vi "改动项处理模块.vi"(6 "执行模式":enum16{"连接模式", "离线模式"}(ring), 7 "改动项 i":T2, 9 "串口配置":T1, 10 "探头属性 i":T7, 11 "TCP ID i":refnum<k5>) -> (0 "error out":errorcluster, 2 "探头属性 o":T7, 3 "TCP ID o":refnum<k5>, 5 "改动项复位 o":T2)   [LabVIEW 2017]
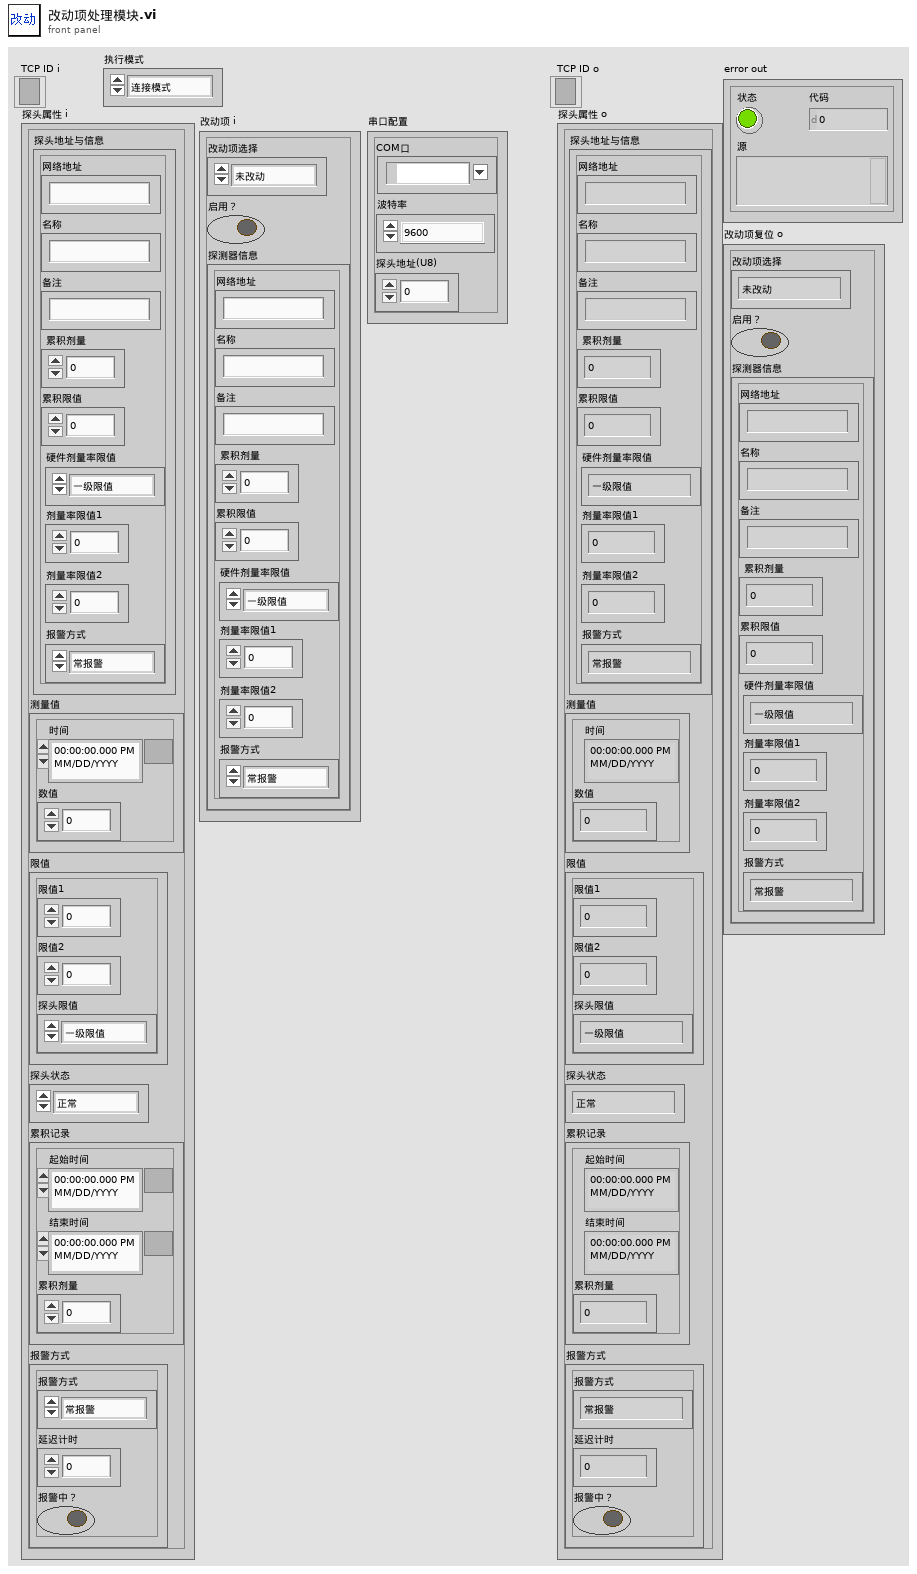
[diagram p1: front panel]
types:
  T1 = typedef "串口配置.ctl" = cluster{"COM口":refnum<visa-resource-name>, "波特率":enum16{"9600", "19200"}, "探头地址(U8)":u8}
  T2 = typedef "改动项.ctl" = cluster{"改动项选择":T3, "启用？":bool, "探测器信息":T4}
  T3 = typedef "改动项选择.ctl" = enum16{"未改动", "改动-启用状态", "改动-探头信息", "改动-报警限值", "动作-手动静音", "动作-重启累积时段", "动作-累积删除", "动作-重连"}
  T4 = typedef "探测器信息.ctl" = cluster{"网络地址":string, "名称":string, "备注":string, "累积剂量":dbl, "累积限值":dbl, "硬件剂量率限值":T5, "剂量率限值1":dbl, "剂量率限值2":dbl, "报警方式":T6}
  T5 = typedef "探头剂量率限值选择.ctl" = enum16{"一级限值", "二级限值"}
  T6 = typedef "报警方式选择.ctl" = enum16{"常报警", "自动静音", "手动静音"}
  T7 = typedef "探头属性.ctl" = cluster{"探头地址与信息":T4, "测量值":T8, "限值":T9, "探头状态":T10, "累积记录":T11, "报警方式":T12}
  T8 = typedef "测量值.ctl" = cluster{"时间":timestamp, "数值":dbl}
  T9 = typedef "剂量率限值.ctl" = cluster{"限值1":dbl, "限值2":dbl, "探头限值":T5}
  T10 = typedef "探头状态.ctl" = enum16{"正常", "离线", "禁用", "一级报警", "二级报警", "累积报警"}
  T11 = typedef "单条累积记录.ctl" = cluster{"起始时间":timestamp, "结束时间":timestamp, "累积剂量":dbl}
  T12 = typedef "报警方式.ctl" = cluster{"报警方式":T6, "延迟计时":u16, "报警中？":bool}
  T13 = typedef "串口模块输入.ctl" = cluster{"串口动作类型":T14, "串口配置":T1, "数据输入":variant}
  T14 = typedef "串口动作类型.ctl" = enum16{"读测量值", "设置报警值", "设置地址", "设置系数", "广播修改波特率", "关闭串口"}
  T15 = typedef "DB动作与数据.ctl" = cluster{"动作类型":T16, "输入数据":variant}
  T16 = typedef "DB动作类型.ctl" = enum16{"DB-文件初始化+连接", "DB-断开连接", "DB-结构初始化", "DB-加载设备", "DB-检查连接状态", "设备-登记新设备+数据表", "设备-删除设备", "设备-修改网址", "设备-修改名称+转移数据", "设备-修改备注", "设备-修改限值", "设备-累积校准", "设备-重排", "数据-获取全部", "数据-删除数据", "数据-写改累积记录+改累积剂量", "读变量-全部设备"}
  T17 = typedef "设备改名卡.ctl" = cluster{"原名":string, "新名":string}
  T18 = typedef "修改网址.ctl" = cluster{"探头属性":T4, "新网址":string}
  T19 = typedef "删除记录输入.ctl" = cluster{"名称":string, "多条记录(空则全删)":T11[]}
  T20 = cluster{"网络地址":bool, "名称":bool, "备注":bool, "累积剂量":bool, "累积限值":bool, "硬件剂量率限值":bool, "剂量率限值1":bool, "剂量率限值2":bool, "报警方式":bool}
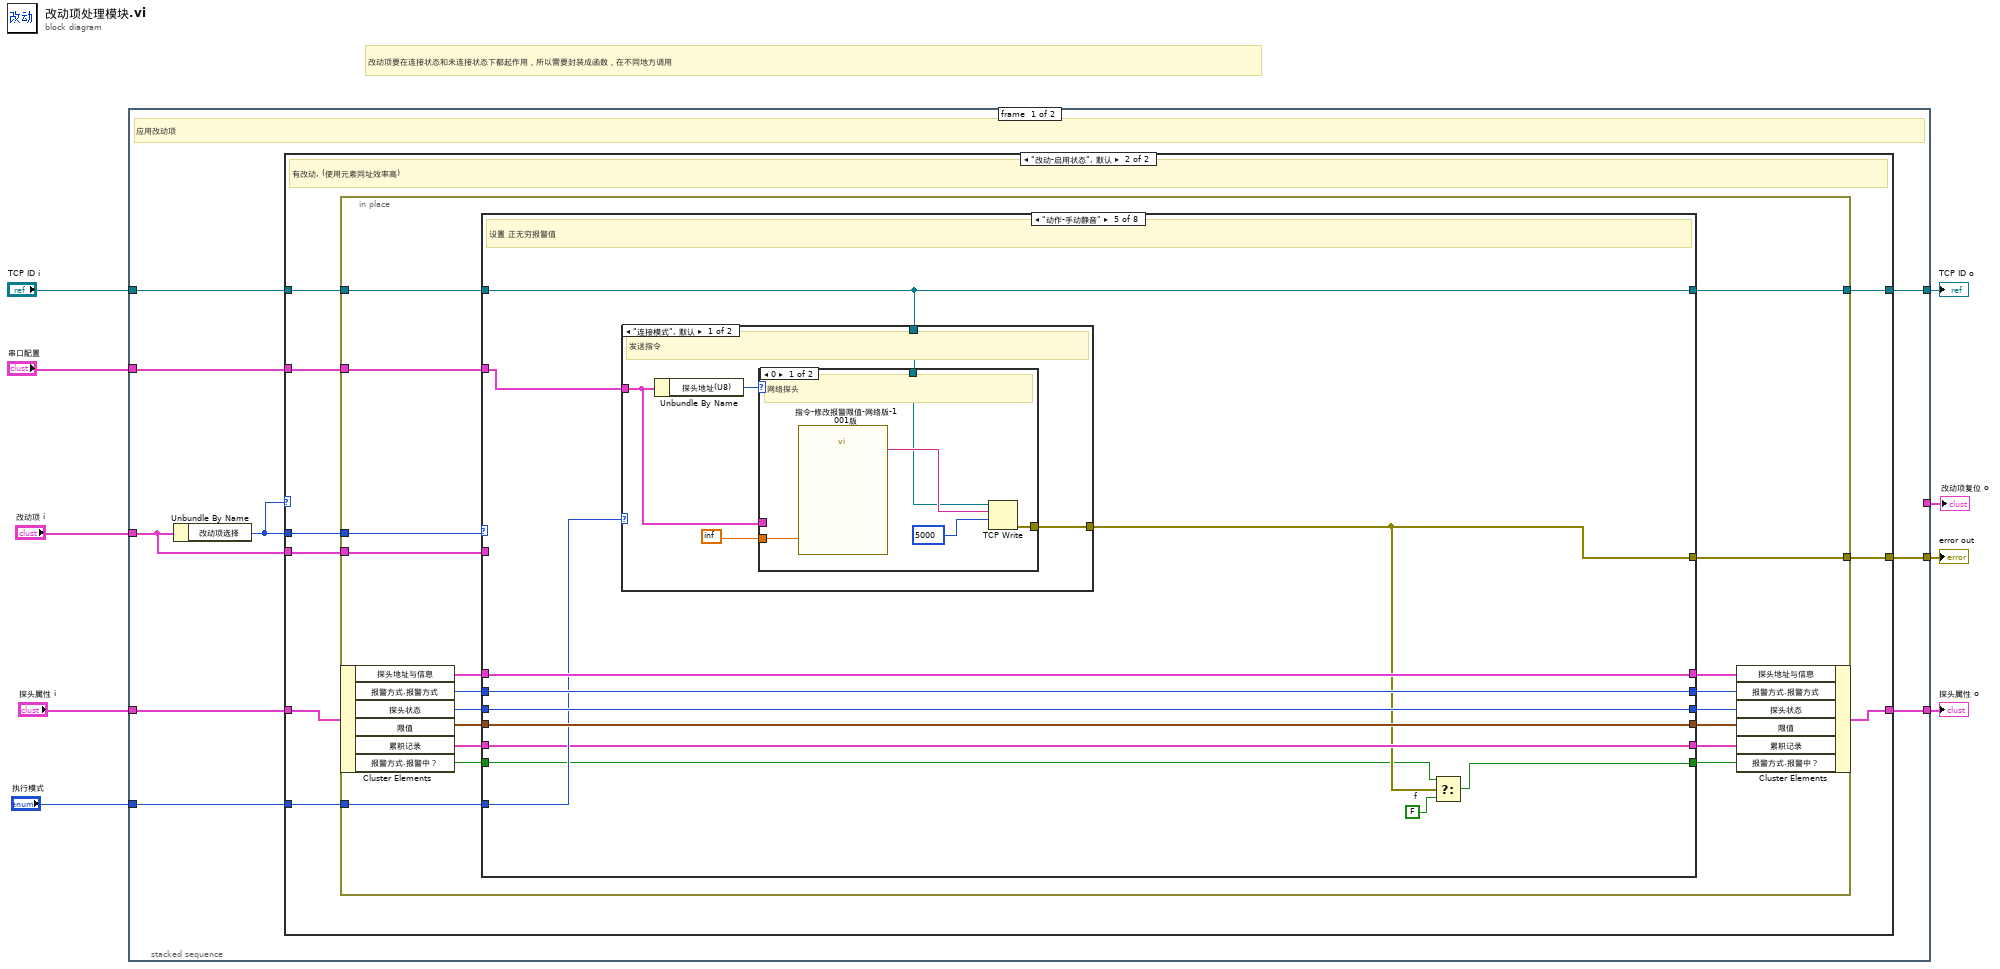
[diagram p0: block diagram]
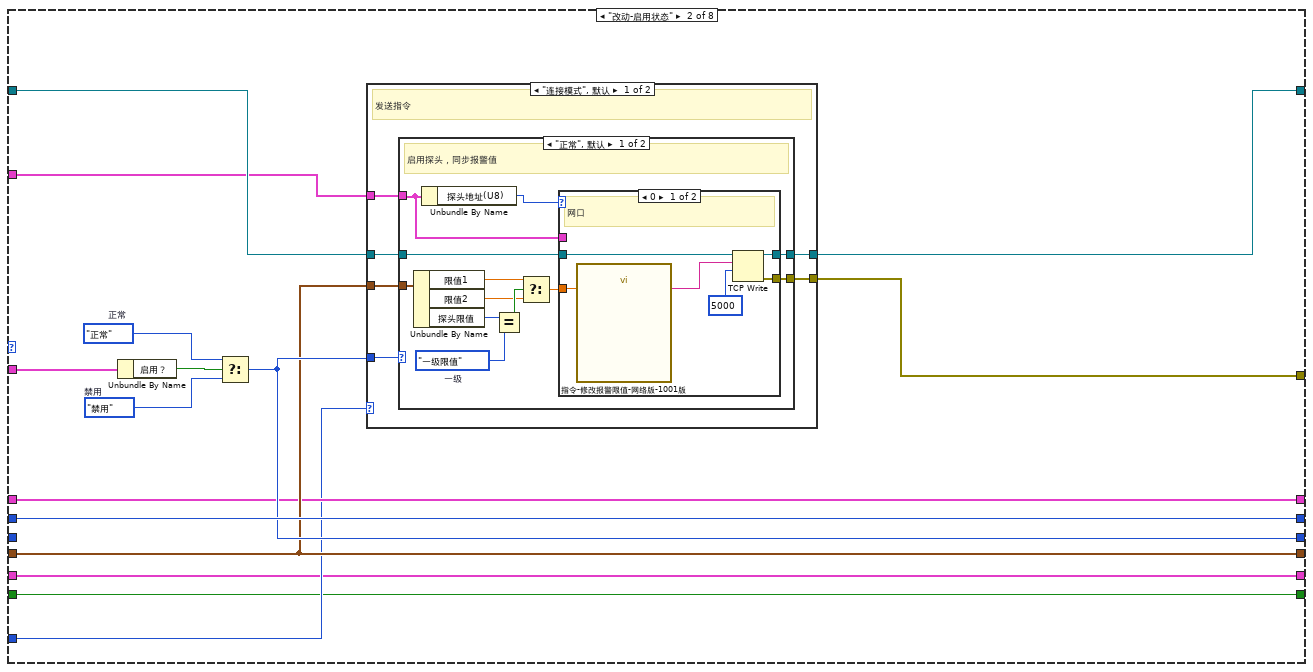
[diagram p4: hidden frame]
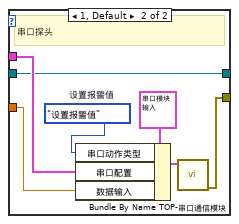
[diagram p5: hidden frame]
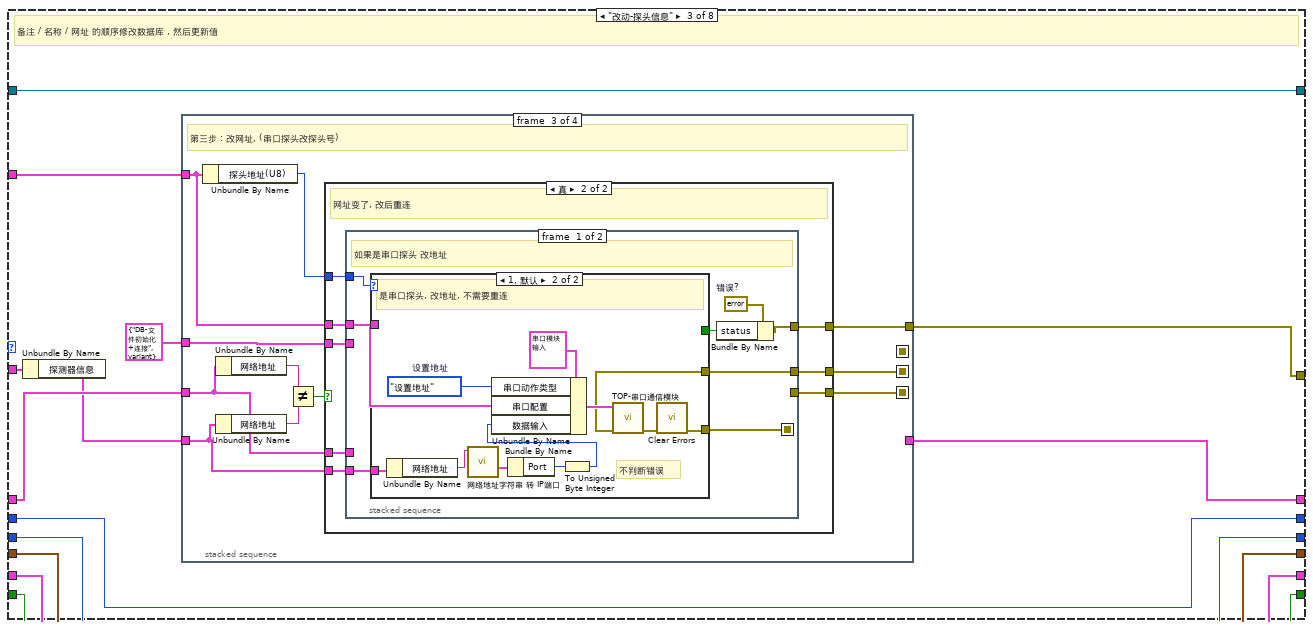
[diagram p8: hidden frame]
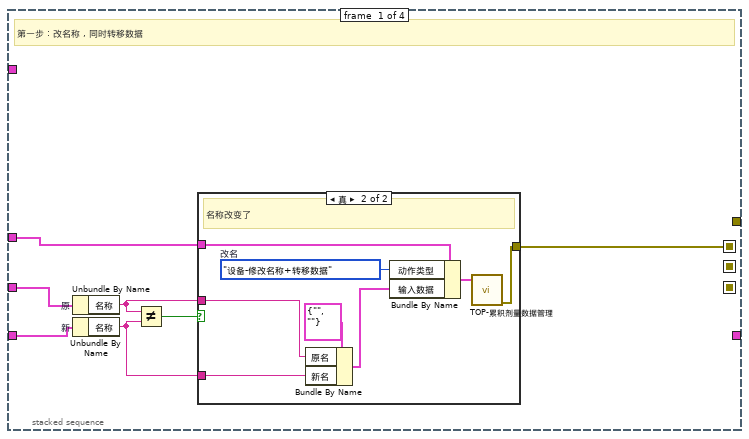
[diagram p9: hidden frame]
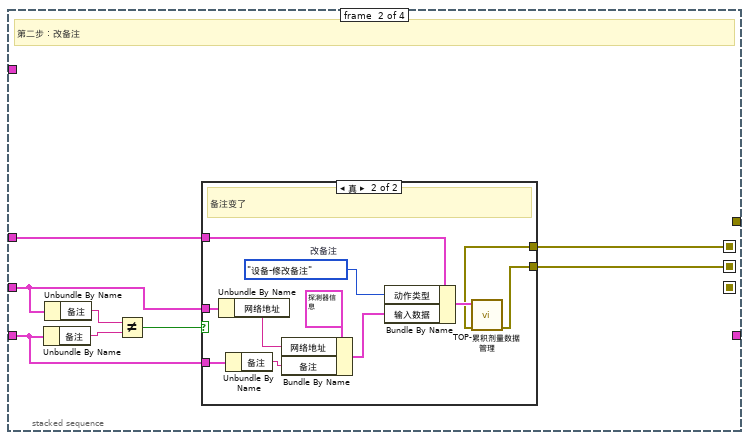
[diagram p11: hidden frame]
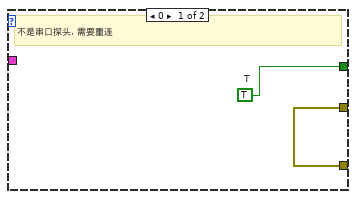
[diagram p14: hidden frame]
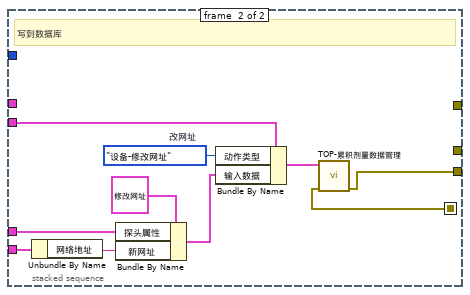
[diagram p15: hidden frame]
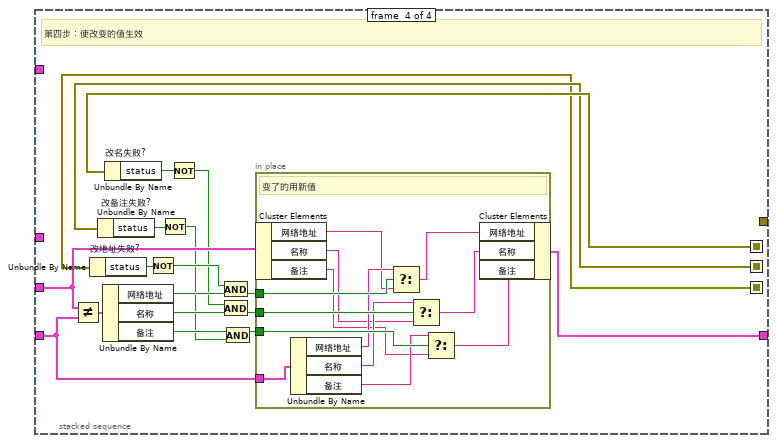
[diagram p16: hidden frame]
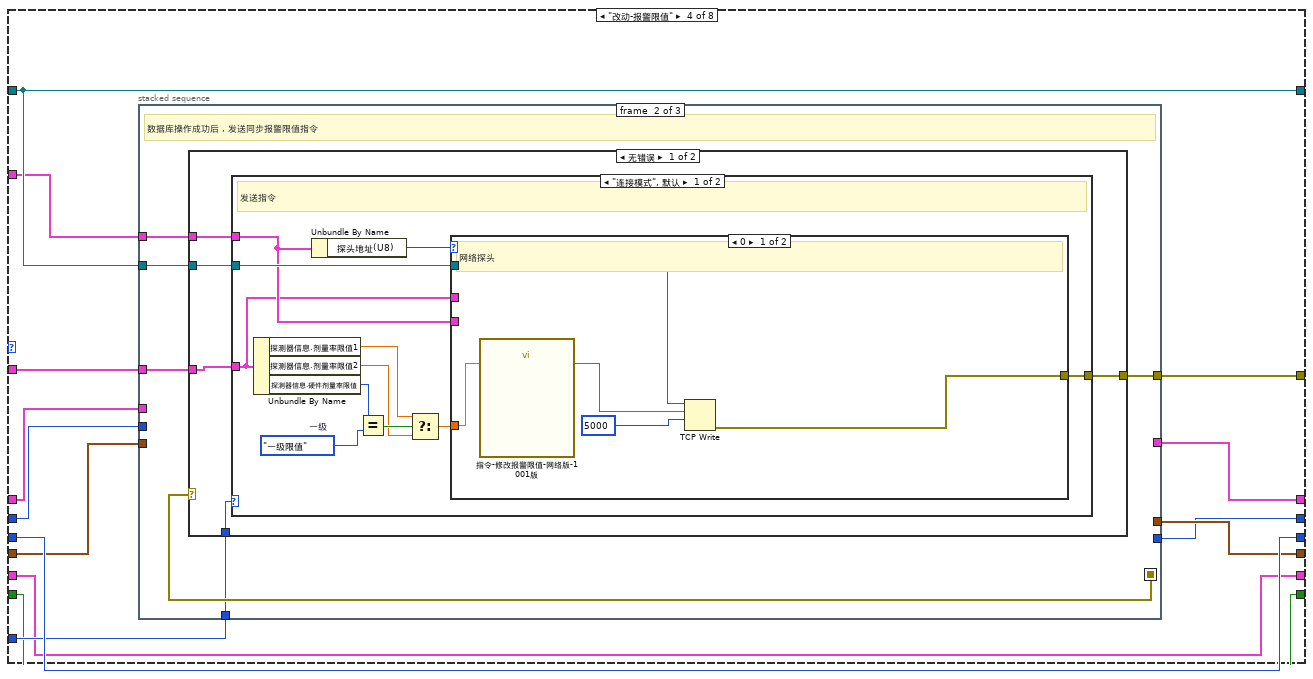
[diagram p17: hidden frame]
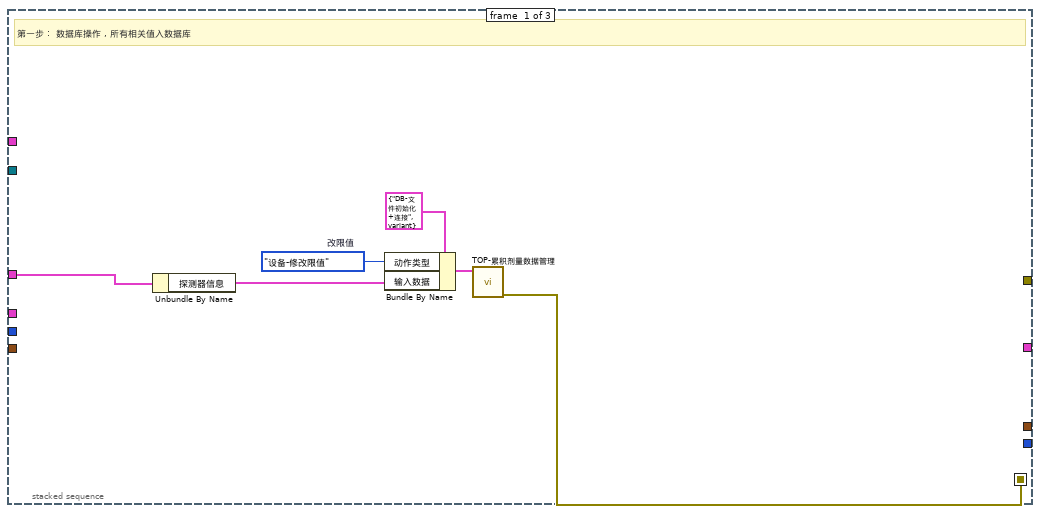
[diagram p18: hidden frame]
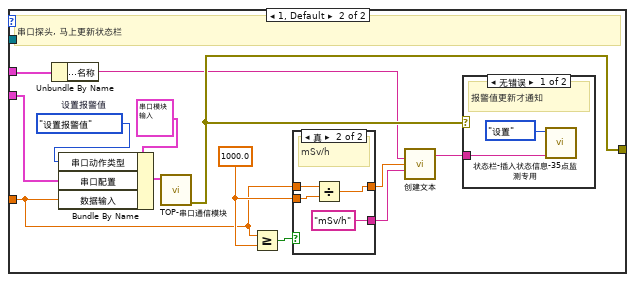
[diagram p19: hidden frame]
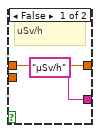
[diagram p20: hidden frame]
diagram:
  # "改动项要在连接状态和未连接状态下都起作用，所以需要封装成函数，在不同地方调用"
  n1 = stacked-sequence {
    tunnel: "改动项 i" -> [w12 _]
    tunnel: [w18 _] -> w5
    tunnel: "探头属性 i" -> [w17 _]
    tunnel: "TCP ID i" -> [w16 _]
    tunnel: [w15 _] -> w4
    tunnel: [w14 _] -> w7
    tunnel: [_ T2 {"改动项选择"=enum."未改动", "启用？"=FALSE, "探测器信息"={"网络地址"="", "名称"="", "备注"="", "累积剂量"=0.0, "累积限值"=0.0, "硬件剂量率限值"=enum."一级限值", "剂量率限值1"=0.0, "剂量率限值2"=0.0, "报警方式"=enum."常报警"}} ("改动项")] -> w3
    tunnel: "执行模式" -> [w13 _]
    tunnel: "串口配置" -> [w10 _]
    frame #0 {
      # "应用改动项"
      n2 = Unbundle By Name(w12) -> ("改动项选择"=w11:T3)
      n3 = case shown="\"改动-启用状态\", 默认" w11 {
        tunnel: w11 -> [_ w29]
        tunnel: [w19 w28] -> w18
        tunnel: w17 -> [w19 w27]
        tunnel: w16 -> [w20 w26]
        tunnel: [_ w25] -> w15
        tunnel: [w20 w24] -> w14
        tunnel: w13 -> [_ w23]
        tunnel: w12 -> [_ w22]
        tunnel: w10 -> [_ w21]
        frame "未改动" {
          # "未改动就不操作"
        }
        frame "改动-启用状态", Default {
          # "有改动, (使用元素同址效率高)"
          n4 = in-place {
            in-place-border: w29 -> [w48]
            in-place-border: w26 -> [w41]
            in-place-border: [w40] -> w24
            in-place-border: [w39] -> w25
            in-place-border: w23 -> [w36]
            in-place-border: w22 -> [w32]
            in-place-border: w21 -> [w33]
            n5 = in-place-cluster #1(w27) -> ("探头地址与信息"=w37:T4, "报警方式.报警方式"=w46:T6, "探头状态"=w45:T10, "限值"=w43:T9, "累积记录"=w35:T11, "报警方式.报警中？"=w31:bool)
            n6 = case shown="\"动作-手动静音\"" w48 {
              tunnel: w32 -> [_ w70 w116 w248 _ _ w382 _]
              tunnel: [w55 w66 w108 w242 w342 w369 w378 w404] -> w47
              tunnel: w46 -> [w55 w66 w108 w240 w342 w369 w378 w404]
              tunnel: [w54 w65 w113 w249 w343 w368 w379 w403] -> w44
              tunnel: w45 -> [w54 _ w113 w249 w343 w368 w379 w403]
              tunnel: w43 -> [w53 w62 w114 w245 w344 w367 w380 w402]
              tunnel: [w53 w62 w114 w243 w344 w367 w380 w402] -> w42
              tunnel: w41 -> [w52 w64 w112 w247 w340 w366 w386 w400]
              tunnel: [w52 w63 w112 w247 w340 w366 w386 w400] -> w40
              tunnel: [_ w57 w107 w246 w335 _ _ w407] -> w39
              tunnel: [w51 w61 w109 w241 w341 w370 w385 w405] -> w38
              tunnel: w37 -> [w51 w61 w115 w244 w341 w370 w372 w405]
              tunnel: w36 -> [_ w60 _ w239 w339 _ _ _]
              tunnel: w35 -> [w50 w59 w106 w238 w338 w365 w375 w401]
              tunnel: [w50 w59 w106 w238 w338 w362 w374 w401] -> w34
              tunnel: w33 -> [_ w58 w105 w237 w337 _ _ _]
              tunnel: w31 -> [w49 w56 w104 w236 w334 w361 w371 w399]
              tunnel: [w49 w56 w104 w236 w333 w361 w371 w399] -> w30
              frame "未改动", Default {
                # "未改动"
              }
              frame "改动-启用状态" {
                w68 = 探头状态."禁用"  # 禁用
                w67 = 探头状态."正常"  # 正常
                n7 = Unbundle By Name(w70) -> ("启用？"=w69:bool)
                n8 = Select(t=w67, s=w69, f=w68) -> (s? t:f=w65:T10)
                n9 = case shown="\"连接模式\", 默认" w60 {
                  tunnel: w65 -> [w76 _]
                  tunnel: w64 -> [w75 w103]
                  tunnel: [w74 w103] -> w63
                  tunnel: w62 -> [w73 _]
                  tunnel: [w72 _] -> w57
                  tunnel: w58 -> [w71 _]
                  frame "连接模式", Default {
                    # "发送指令"
                    n10 = case shown="\"正常\", 默认" w76 {
                      tunnel: w73 -> [w88 _]
                      tunnel: w75 -> [w87 w102]
                      tunnel: [w86 w102] -> w74
                      tunnel: [w85 _] -> w72
                      tunnel: w71 -> [w77 _]
                      frame "正常", Default {
                        w83 = 探头剂量率限值选择."一级限值"  # 一级
                        # "启用探头，同步报警值"
                        n11 = Unbundle By Name(w88) -> ("限值1"=w80:dbl, "限值2"=w81:dbl, "探头限值"=w84:T5)
                        n12 = Unbundle By Name(w77) -> ("探头地址(U8)"=w78:u8)
                        n13 = Equal?(x=w84, y=w83) -> (x = y?=w82:bool)
                        n14 = Select(t=w80, s=w82, f=w81) -> (s? t:f=w79:dbl)
                        n15 = case shown="0" w78 {
                          tunnel: w87 -> [w92 w95]
                          tunnel: [w91 w95] -> w86
                          tunnel: [w90 w96] -> w85
                          tunnel: w79 -> [w89 w97]
                          tunnel: w77 -> [_ w98]
                          frame 0 {
                            # "网口"
                            n16 = call "指令-修改报警限值-网络版-1001版.vi"("限值"=w89) -> ("指令输出"=w93:string)  [unwired: 10 in]
                            n17 = TCP Write(connection ID=w92, data in=w93, 9:5000 ("超时毫秒(25000)")) -> (connection ID out=w91:refnum<k5>, error out=w90:errorcluster)  [unwired: 1 in, 1 out]
                          }
                          frame 1, Default {
                            w101 = 串口动作类型."设置报警值"  # 设置报警值
                            # "串口探头"
                            n18 = Bundle By Name(cluster=T13 {"串口动作类型"=enum."读测量值", "串口配置"={"COM口"="", "波特率"=enum."9600", "探头地址(U8)"=0}, "数据输入"=variant} ("串口模块输入"), "串口动作类型"=w101, "串口配置"=w98, "数据输入"=w97) -> (w100:T13)
                            n19 = call "TOP-串口通信模块.vi"("串口模块输入"=w100) -> ("error out"=w96:errorcluster)  [unwired: 9 in, 1 out]
                          }
                        }
                      }
                      frame "禁用" {
                      }
                    }
                  }
                  frame "离线模式" {
                    # "不发送指令"
                  }
                }
              }
              frame "改动-探头信息" {
                # "备注 / 名称 / 网址 的顺序修改数据库 , 然后更新值"
                n20 = Unbundle By Name(w116) -> ("探测器信息"=w110:T4)
                n21 = stacked-sequence {
                  seq-local: [w122 _ _ _] -> [_ w137 _ w212]
                  seq-local: [_ w138 _ _] -> [_ _ w161 w211]
                  seq-local: [_ _ w155 _] -> [_ _ _ w210]
                  tunnel: w115 -> [w121 w136 w160 w221]
                  tunnel: T15 {"动作类型"=enum."DB-文件初始化+连接", "输入数据"=variant} ("DB动作集") -> [w123 w139 w162 _]
                  tunnel: w110 -> [w120 w135 w159 w217]
                  tunnel: [_ _ _ w216] -> w109
                  tunnel: [_ _ w154 _] -> w107
                  tunnel: w105 -> [_ _ w152 _]
                  frame #0 {
                    # "第一步 : 改名称 , 同时转移数据"
                    n22 = Unbundle By Name "原"(w121) -> ("名称"=w118:string)
                    n23 = Unbundle By Name "新"(w120) -> ("名称"=w117:string)
                    n24 = Not Equal?(x=w118, y=w117) -> (x != y?=w119:bool)
                    n25 = case shown="真" w119 {
                      tunnel: w123 -> [_ w131]
                      tunnel: [_ w126] -> w122
                      tunnel: w118 -> [_ w125]
                      tunnel: w117 -> [_ w124]
                      frame False {
                        # "名称没变"
                      }
                      frame True {
                        w130 = DB动作类型."设备-修改名称+转移数据"  # 改名
                        # "名称改变了"
                        n26 = Bundle By Name(cluster=T17 {"原名"="", "新名"=""} ("改名"), "原名"=w125, "新名"=w124) -> (w128:T17)
                        n27 = Bundle By Name(cluster=w131, "动作类型"=w130, "输入数据"=w128) -> (w127:T15)
                        n28 = call "TOP-累积剂量数据管理.vi"("DB动作集"=w127) -> ("error out"=w126:errorcluster)  [unwired: 9 in, 1 out]
                      }
                    }
                  }
                  frame #1 {
                    # "第二步 : 改备注"
                    n29 = Unbundle By Name(w135) -> ("备注"=w133:string)
                    n30 = Unbundle By Name(w136) -> ("备注"=w134:string)
                    n31 = Not Equal?(x=w134, y=w133) -> (x != y?=w132:bool)
                    n32 = case shown="真" w132 {
                      tunnel: w139 -> [_ w150]
                      tunnel: [w140 w144] -> w138
                      tunnel: w137 -> [w140 w143]
                      tunnel: w136 -> [_ w142]
                      tunnel: w135 -> [_ w141]
                      frame False {
                        # "备注没变"
                      }
                      frame True {
                        w151 = DB动作类型."设备-修改备注"  # 改备注
                        # "备注变了"
                        n33 = Unbundle By Name(w142) -> ("网络地址"=w147:string)
                        n34 = Unbundle By Name(w141) -> ("备注"=w148:string)
                        n35 = Bundle By Name(cluster=T4 {"网络地址"="", "名称"="", "备注"="", "累积剂量"=0.0, "累积限值"=0.0, "硬件剂量率限值"=enum."一级限值", "剂量率限值1"=0.0, "剂量率限值2"=0.0, "报警方式"=enum."常报警"} ("探测器信息-改备注"), "网络地址"=w147, "备注"=w148) -> (w146:T4)
                        n36 = Bundle By Name(cluster=w150, "动作类型"=w151, "输入数据"=w146) -> (w145:T15)
                        n37 = call "TOP-累积剂量数据管理.vi"("错误输出"=w143, "DB动作集"=w145) -> ("error out"=w144:errorcluster)  [unwired: 8 in, 1 out]
                      }
                    }
                  }
                  frame #2 {
                    # "第三步 : 改网址, (串口探头改探头号)"
                    n38 = Unbundle By Name(w152) -> ("探头地址(U8)"=w153:u8)
                    n39 = Unbundle By Name(w160) -> ("网络地址"=w158:string)
                    n40 = Unbundle By Name(w159) -> ("网络地址"=w157:string)
                    n41 = Not Equal?(x=w158, y=w157) -> (x != y?=w156:bool)
                    n42 = case shown="真" w156 {
                      tunnel: w162 -> [_ w167]
                      tunnel: w161 -> [w163 w171]
                      tunnel: w160 -> [_ w170]
                      tunnel: w159 -> [_ w169]
                      tunnel: [w163 w168] -> w155
                      tunnel: [_ w166] -> w154
                      tunnel: w153 -> [_ w165]
                      tunnel: w152 -> [_ w164]
                      frame False {
                        # "网址没变"
                      }
                      frame True {
                        # "网址变了, 改后重连"
                        n43 = stacked-sequence {
                          seq-local: [w172 _] -> [_ w194]
                          tunnel: w171 -> [w173 _]
                          tunnel: w170 -> [_ w198]
                          tunnel: w169 -> [w177 w197]
                          tunnel: [_ w196] -> w168
                          tunnel: w167 -> [_ w195]
                          tunnel: [w175 _] -> w166
                          tunnel: w165 -> [w179 _]
                          tunnel: w164 -> [w178 _]
                          frame #0 {
                            w176 = errorcluster {"status"=TRUE, "code"=0, "source"=""}  # 错误?
                            # "如果是串口探头 改地址"
                            n44 = case shown="1, 默认" w179 {
                              tunnel: w178 -> [_ w186]
                              tunnel: w177 -> [_ w191]
                              tunnel: [w181 _] -> w174
                              tunnel: w173 -> [w180 w184]
                              tunnel: [w180 w182] -> w172
                              frame 0 {
                                w181 = TRUE  # T
                                # "不是串口探头, 需要重连"
                              }
                              frame 1, Default {
                                w192 = 串口动作类型."设置地址"  # 设置地址
                                # "不判断错误"
                                # "是串口探头, 改地址, 不需要重连"
                                n45 = Unbundle By Name(w191) -> ("网络地址"=w189:string)
                                n46 = call "网络地址字符串 转 IP端口.vi"("IP端口字符串"=w189) -> ("IP端口"=w190:cluster{"IP":string, "Port":u16})  [unwired: 10 in]
                                n47 = Unbundle By Name(w190) -> ("Port"=w188:u16)
                                n48 = To Unsigned Byte Integer(number=w188) -> (unsigned 8bit integer=w187:u8)
                                n49 = Bundle By Name(cluster=T13 {"串口动作类型"=enum."读测量值", "串口配置"={"COM口"="", "波特率"=enum."9600", "探头地址(U8)"=0}, "数据输入"=variant} ("串口模块输入"), "串口动作类型"=w192, "串口配置"=w186, "数据输入"=w187) -> (w185:T13)
                                n50 = call "TOP-串口通信模块.vi"("错误输入（无错误）"=w184, "串口模块输入"=w185) -> ("error out"=w183:errorcluster)  [unwired: 8 in, 1 out]
                                n51 = call <vilib>:"Clear Errors.vi"("error in (no error)"=w183) -> ("error out"=w182:errorcluster)  [unwired: 5 in, 1 out]
                              }
                            }
                            n52 = Bundle By Name(cluster=w176, "status"=w174) -> (w175:errorcluster)
                          }
                          frame #1 {
                            w203 = DB动作类型."设备-修改网址"  # 改网址
                            # "写到数据库"
                            n53 = Unbundle By Name(w197) -> ("网络地址"=w201:string)
                            n54 = Bundle By Name(cluster=T18 {"探头属性"={"网络地址"="", "名称"="", "备注"="", "累积剂量"=0.0, "累积限值"=0.0, "硬件剂量率限值"=enum."一级限值", "剂量率限值1"=0.0, "剂量率限值2"=0.0, "报警方式"=enum."常报警"}, "新网址"=""} ("类型"), "探头属性"=w198, "新网址"=w201) -> (w200:T18)
                            n55 = Bundle By Name(cluster=w195, "动作类型"=w203, "输入数据"=w200) -> (w199:T15)
                            n56 = call "TOP-累积剂量数据管理.vi"("错误输出"=w194, "DB动作集"=w199) -> ("error out"=w196:errorcluster)  [unwired: 8 in, 1 out]
                          }
                        }
                      }
                    }
                  }
                  frame #3 {
                    # "第四步 : 使改变的值生效"
                    n57 = Not Equal?(x=w221, y=w217) -> (x != y?=w222:T20)
                    n58 = Unbundle By Name "改地址失败?"(w210) -> ("status"=w207:bool)
                    n59 = Unbundle By Name "改备注失败?"(w211) -> ("status"=w208:bool)
                    n60 = Unbundle By Name(w222) -> ("网络地址"=w220:bool, "名称"=w219:bool, "备注"=w218:bool)
                    n61 = Unbundle By Name "改名失败?"(w212) -> ("status"=w209:bool)
                    n62 = Not(x=w207) -> (.not. x?=w206:bool)
                    n63 = Not(x=w208) -> (.not. x?=w204:bool)
                    n64 = Not(x=w209) -> (.not. x?=w205:bool)
                    n65 = And(x=w206, y=w220) -> (x .and. y?=w215:bool)
                    n66 = And(x=w205, y=w219) -> (x .and. y?=w214:bool)
                    n67 = And(x=w218, y=w204) -> (x .and. y?=w213:bool)
                    n68 = in-place {
                      in-place-border: w215 -> [w235]
                      in-place-border: w214 -> [w234]
                      in-place-border: w213 -> [w233]
                      in-place-border: w217 -> [w232]
                      # "变了的用新值"
                      n69 = in-place-cluster #2(w221) -> ("网络地址"=w228:string, "名称"=w227:string, "备注"=w226:string)
                      n70 = Unbundle By Name(w232) -> ("网络地址"=w231:string, "名称"=w230:string, "备注"=w229:string)
                      n71 = Select(t=w231, s=w235, f=w228) -> (s? t:f=w225:string)
                      n72 = Select(t=w230, s=w234, f=w227) -> (s? t:f=w224:string)
                      n73 = Select(t=w229, s=w233, f=w226) -> (s? t:f=w223:string)
                      n74 = in-place-cluster #2("网络地址"=w225, "名称"=w224, "备注"=w223) -> (w216:T4)
                    }
                  }
                }
              }
              frame "改动-报警限值" {
                n75 = stacked-sequence {
                  seq-local: [w250 _ _] -> [_ w261 w311]
                  tunnel: w248 -> [w252 w260 w310]
                  tunnel: w247 -> [_ w259 _]
                  tunnel: [_ w258 _] -> w246
                  tunnel: w245 -> [_ _ w309]
                  tunnel: w244 -> [_ _ w308]
                  tunnel: [_ _ w307] -> w243
                  tunnel: [_ _ w306] -> w242
                  tunnel: [_ _ w305] -> w241
                  tunnel: w240 -> [_ _ w304]
                  tunnel: w239 -> [_ w257 _]
                  tunnel: w237 -> [_ w256 _]
                  frame #0 {
                    w255 = DB动作类型."设备-修改限值"  # 改限值
                    # "第一步 :  数据库操作 , 所有相关值入数据库"
                    n76 = Unbundle By Name(w252) -> ("探测器信息"=w251:T4)
                    n77 = Bundle By Name(cluster=T15 {"动作类型"=enum."DB-文件初始化+连接", "输入数据"=variant} ("DB动作集"), "动作类型"=w255, "输入数据"=w251) -> (w254:T15)
                    n78 = call "TOP-累积剂量数据管理.vi"("DB动作集"=w254) -> ("error out"=w250:errorcluster)  [unwired: 9 in, 1 out]
                  }
                  frame #1 {
                    # "数据库操作成功后 , 发送同步报警限值指令"
                    n79 = case shown="无错误" w261 {
                      tunnel: w260 -> [w266 _]
                      tunnel: w259 -> [w265 _]
                      tunnel: [w264 _] -> w258
                      tunnel: w257 -> [w263 _]
                      tunnel: w256 -> [w262 _]
                      frame No Error {
                        n80 = case shown="\"连接模式\", 默认" w263 {
                          tunnel: w266 -> [w267 _]
                          tunnel: w265 -> [w271 _]
                          tunnel: [w270 _] -> w264
                          tunnel: w262 -> [w268 _]
                          frame "连接模式", Default {
                            w276 = 探头剂量率限值选择."一级限值"  # 一级
                            # "发送指令"
                            n81 = Unbundle By Name(w267) -> ("探测器信息.剂量率限值1"=w274:dbl, "探测器信息.剂量率限值2"=w273:dbl, "探测器信息.硬件剂量率限值"=w277:T5)
                            n82 = Unbundle By Name(w268) -> ("探头地址(U8)"=w269:u8)
                            n83 = Equal?(x=w277, y=w276) -> (x = y?=w275:bool)
                            n84 = Select(t=w274, s=w275, f=w273) -> (s? t:f=w272:dbl)
                            n85 = case shown="0" w269 {
                              tunnel: w272 -> [w280 w285]
                              tunnel: w271 -> [w279 _]
                              tunnel: [w278 w290] -> w270
                              tunnel: w268 -> [_ w292]
                              tunnel: w267 -> [_ w289]
                              frame 0 {
                                # "网络探头"
                                n86 = call "指令-修改报警限值-网络版-1001版.vi"("限值"=w280) -> ("指令输出"=w282:string)  [unwired: 10 in]
                                n87 = TCP Write(connection ID=w279, data in=w282, 9:5000 ("超时毫秒(25000)")) -> (error out=w278:errorcluster)  [unwired: 1 in, 2 out]
                              }
                              frame 1, Default {
                                w286 = 1000.0 ("y")
                                w293 = 串口动作类型."设置报警值"  # 设置报警值
                                # "串口探头, 马上更新状态栏"
                                n88 = Unbundle By Name(w289) -> ("探测器信息.名称"=w288:string)
                                n89 = Bundle By Name(cluster=T13 {"串口动作类型"=enum."读测量值", "串口配置"={"COM口"="", "波特率"=enum."9600", "探头地址(U8)"=0}, "数据输入"=variant} ("串口模块输入"), "串口动作类型"=w293, "串口配置"=w292, "数据输入"=w285) -> (w295:T13)
                                n90 = call "TOP-串口通信模块.vi"("串口模块输入"=w295) -> ("error out"=w290:errorcluster)  [unwired: 9 in, 1 out]
                                n91 = Greater Or Equal?(x=w285, y=w286) -> (x >= y?=w287:bool)
                                n92 = case shown="真" w287 {
                                tunnel: [w297 w299] -> w284
                                tunnel: w285 -> [w297 w300]
                                tunnel: ["μSv/h" ("单位") "mSv/h" ("单位")] -> w283
                                tunnel: w286 -> [_ w298]
                                frame False {
                                # "uSv/h"
                                }
                                frame True {
                                # "mSv/h"
                                n93 = Divide(x=w300, y=w298) -> (x/y=w299:dbl)
                                }
                                }
                                n94 = call "创建文本"("探头名称"=w288, "限值"=w284, "单位"=w283) -> ("Result"=w291:string)  [unwired: 11 in, 1 out]
                                n95 = case shown="无错误" w290 {
                                tunnel: w291 -> [w302 _]
                                frame No Error {
                                # "报警值更新才通知"
                                n96 = call "状态栏-插入状态信息-35点监测专用.vi"("消息内容"=w302, "状态类型"=enum16{"全部", "报警", "通信", "设置"}."设置") -> ()  [unwired: 10 in]
                                }
                                frame Error {
                                }
                                }
                              }
                            }
                          }
                          frame "离线模式" {
                            # "不发送指令"
                          }
                        }
                      }
                      frame Error {
                        # "DB错误不算通信错误"
                      }
                    }
                  }
                  frame #2 {
                    # "只要数据库操作没出错就先使属性生效, \n这样即使离线模式也能修改限值,"
                    # "使值生效"
                    n97 = case shown="无错误" w311 {
                      tunnel: w310 -> [w318 w332]
                      tunnel: w309 -> [w316 w330]
                      tunnel: w308 -> [w317 _]
                      tunnel: [w314 w330] -> w307
                      tunnel: [w313 w329] -> w306
                      tunnel: [w312 w331] -> w305
                      tunnel: w304 -> [_ w329]
                      frame No Error {
                        n98 = Unbundle By Name(w318) -> ("探测器信息"=w315:T4)
                        n99 = in-place {
                          in-place-border: w317 -> [w328]
                          in-place-border: w315 -> [w323]
                          in-place-border: [w319] -> w313
                          n100 = in-place-cluster #3(w315) -> ()  [unwired: 4 out]
                          n101 = in-place-cluster #4(w316) -> ()  [unwired: 3 out]
                          n102 = Unbundle By Name(w323) -> ("剂量率限值1"=w322:dbl, "剂量率限值2"=w321:dbl, "硬件剂量率限值"=w320:T5, "报警方式"=w319:T6)
                          n103 = Unbundle By Name "保留原信息"(w328) -> ("网络地址"=w327:string, "名称"=w326:string, "备注"=w325:string, "累积剂量"=w324:dbl)
                          n104 = in-place-cluster #3("网络地址"=w327, "名称"=w326, "备注"=w325, "累积剂量"=w324) -> (w312:T4)
                          n105 = in-place-cluster #4("限值1"=w322, "限值2"=w321, "探头限值"=w320) -> (w314:T9)
                        }
                      }
                      frame Error {
                        n106 = Unbundle By Name(w332) -> ("探测器信息"=w331:T4)
                      }
                    }
                  }
                }
              }
              frame "动作-手动静音" {
                w336 = FALSE  # f
                # "设置 正无穷报警值"
                n107 = case shown="\"连接模式\", 默认" w339 {
                  tunnel: [w349 _] -> w335
                  tunnel: w340 -> [w347 _]
                  tunnel: w337 -> [w345 _]
                  frame "连接模式", Default {
                    # "发送指令"
                    n108 = Unbundle By Name(w345) -> ("探头地址(U8)"=w346:u8)
                    n109 = case shown="0" w346 {
                      tunnel: [w352 w355] -> w349
                      tunnel: inf -> [w351 w356]
                      tunnel: w347 -> [w350 _]
                      tunnel: w345 -> [_ w357]
                      frame 0 {
                        # "网络探头"
                        n110 = call "指令-修改报警限值-网络版-1001版.vi"("限值"=w351) -> ("指令输出"=w354:string)  [unwired: 10 in]
                        n111 = TCP Write(connection ID=w350, data in=w354, 9:5000 ("超时毫秒(25000)")) -> (error out=w352:errorcluster)  [unwired: 1 in, 2 out]
                      }
                      frame 1, Default {
                        w358 = 串口动作类型."设置报警值"  # 设置报警值
                        # "串口探头"
                        n112 = Bundle By Name(cluster=T13 {"串口动作类型"=enum."读测量值", "串口配置"={"COM口"="", "波特率"=enum."9600", "探头地址(U8)"=0}, "数据输入"=variant} ("串口模块输入"), "串口动作类型"=w358, "串口配置"=w357, "数据输入"=w356) -> (w360:T13)
                        n113 = call "TOP-串口通信模块.vi"("串口模块输入"=w360) -> ("error out"=w355:errorcluster)  [unwired: 9 in, 1 out]
                      }
                    }
                  }
                  frame "离线模式" {
                    # "不发送指令"
                  }
                }
                n114 = Select(t=w334, s=w335, f=w336) -> (s? t:f=w333:bool)
              }
              frame "动作-重启累积时段" {
                # "重新初始化累积记录，达到另起累积时段的效果"
                n115 = Get Date/Time In Seconds() -> (seconds since 1Jan1904=w364:timestamp)
                n116 = Bundle By Name(cluster=w365, "起始时间"=w364, "结束时间"=w364, "累积剂量"=0.0) -> (w362:T11)
              }
              frame "动作-累积删除" {
                # "如果是清空操作, 则需要重启累积,\n否则不用重启"
                # "注意: 清零操作时 返回删除量时正无穷"
                # "这里只改变累积剂量值, 数据库操作不在这里进行, 此操作即使在掉线情况下任然要生效"
                n117 = Unbundle By Name "删除量"(w382) -> ("探测器信息.累积剂量"=w377:dbl)
                n118 = in-place {
                  in-place-border: w377 -> [w398]
                  n119 = in-place-cluster #5(w372) -> ("累积剂量"=w396:dbl)
                  n120 = Subtract(x=w396, y=w398) -> (x-y=w397:dbl)
                  n121 = In Range and Coerce(upper limit=w396, x=w397, lower limit=0.0 ("下限")) -> (coerced(x)=w394:dbl)  [unwired: 1 out]
                  n122 = in-place-cluster #5("累积剂量"=w394) -> (w385:T4)
                }
                n123 = Equal?(x=inf, y=w377) -> (x = y?=w373:bool)
                n124 = case shown="真" w373 {
                  tunnel: w372 -> [_ w388]
                  frame False {
                    # "删除部分数据, 不需要再在数据库上删除数据"
                  }
                  frame True {
                    w391 = DB动作类型."数据-删除数据"  # 删除数据
                    # "清空操作的话, 需要在执行一次删除数据, \n防止上个累积记录残留"
                    n125 = Unbundle By Name(w388) -> ("名称"=w387:string)
                    n126 = Bundle By Name(cluster=T19 {"名称"="", "多条记录(空则全删)"=[]}, "名称"=w387) -> (w389:T19)
                    n127 = Bundle By Name(cluster=T15 {"动作类型"=enum."DB-文件初始化+连接", "输入数据"=variant} ("DB动作集"), "动作类型"=w391, "输入数据"=w389) -> (w392:T15)
                    n128 = call "TOP-累积剂量数据管理.vi"("DB动作集"=w392) -> ()  [unwired: 9 in, 2 out]
                  }
                }
                n129 = Get Date/Time In Seconds() -> (seconds since 1Jan1904=w384:timestamp)
                n130 = Bundle By Name(cluster=w375, "起始时间"=w384, "结束时间"=w384, "累积剂量"=0.0) -> (w381:T11)
                n131 = Select(t=w381, s=w373, f=w375) -> (s? t:f=w374:T11)
              }
              frame "动作-重连" {
                w406 = TRUE  # T
                # "这个动作会导致通信模块 网口模式断开重连 串口模式应用新的单口和波特率"
                n132 = Bundle By Name(cluster=errorcluster {"status"=FALSE, "code"=0, "source"=""} ("error out"), "status"=w406) -> (w407:errorcluster)
              }
            }
            n133 = in-place-cluster #1("探头地址与信息"=w38, "报警方式.报警方式"=w47, "探头状态"=w44, "限值"=w42, "累积记录"=w34, "报警方式.报警中？"=w30) -> (w28:T7)
          }
        }
      }
    }
    frame #1 {
      # "改动项复位"
    }
  }
  "TCP ID o" <- w7
  "探头属性 o" <- w5
  "error out" <- w4
  "改动项复位 o" <- w3
